vi "Verify and Check-In.vi"(0 "Guest Manager Model in":refnum<class "Guest Manager Model.lvclass">, 5 "Room No":string, 7 "Guest Contact Number":string, 9 "Primary Guest Name":string, 11 "error in (no error)":errorcluster, 12 "Adults":u32, 13 "Children":u32) -> (4 "Guest Manager Model out":refnum<class "Guest Manager Model.lvclass">, 15 "error out":errorcluster)   [LabVIEW 2023, in "Guest Manager Model.lvlib" / "Guest Manager Model.lvclass"]
uses:
  Guest Manager Model.lvclass
  Guest Manager Model.lvclass/Guest Manager Model.ctl
  <vilib>/ActorFramework/Actor/Actor.lvclass
  Interfaces/Incoming Rooms Manager Model Interface Messages/Verify and Check-in Msg/Verify and Check-in Msg.lvclass
  C:/Program Files/National Instruments/LabVIEW 2023/vi.lib/ActorFramework/Actor/Actor.lvclass
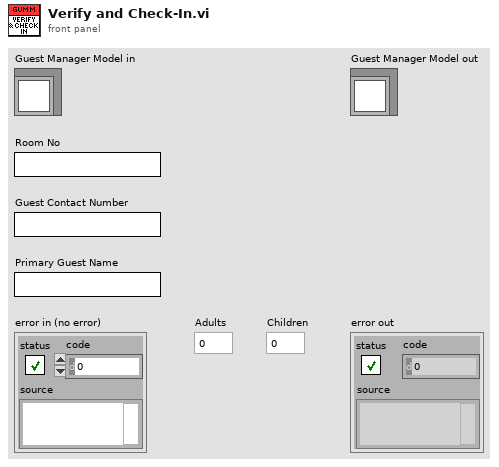
[diagram p1: front panel]
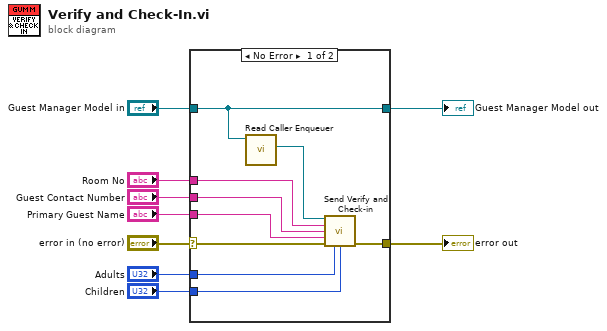
[diagram p0: block diagram]
diagram:
  n1 = case shown="No Error" "error in (no error)" {
    selector: "error in (no error)" -> [w17 w20]
    tunnel: [w16 w20] -> w8
    tunnel: [w18 w19] -> w6
    tunnel: "Guest Manager Model in" -> [w18 w19]
    tunnel: "Room No" -> [w14 _]
    tunnel: "Guest Contact Number" -> [w13 _]
    tunnel: "Primary Guest Name" -> [w12 _]
    tunnel: "Adults" -> [w11 _]
    tunnel: "Children" -> [w10 _]
    frame No Error {
      n2 = call <vilib>:"Read Caller Enqueuer.vi"("Actor"=w18) -> ("Caller Enqueuer"=w15:refnum<class "Message Enqueuer.lvclass">)  [unwired: 10 in]
      n3 = call "Send Verify and Check-in.vi"("Message Enqueuer"=w15, "Room No"=w14, "Guest Contact Number"=w13, "Primary Guest Name"=w12, "error in (no error)"=w17, "Adults"=w11, "Children"=w10) -> ("error out"=w16:errorcluster)  [unwired: 7 in, 1 out]
    }
    frame Error {
    }
  }
  "error out" <- w8
  "Guest Manager Model out" <- w6
